vi "Shooter Simulator.vi"() -> ()   [LabVIEW 2015]
uses:
  Shooter Simulator Sensor Data.ctl
  Shooter Simulator Globals.vi
panel:
  out "R Encoder Rate":dbl
  out "L Encoder Rate":dbl
  in  "reset":bool
  out "Top Limit Switch":bool
  out "Angle Encoder Val":dbl
  out "On Fire":bool
  out "R Motor":dbl(slide) scale=-1.0..1.0
  out "L Motor":dbl(slide) scale=-1.0..1.0
  out "R RPM":dbl(knob) scale=0.0..5000.0
  out "L RPM":dbl(knob) scale=0.0..5000.0
  out "Angle Motor":dbl(slide) scale=-1.0..1.0
  out "Bottom Limit Switch":bool
  in  "Angle":dbl(slide) scale=0.0..90.0
  # "PUT ME IN PERIODIC TASKS"
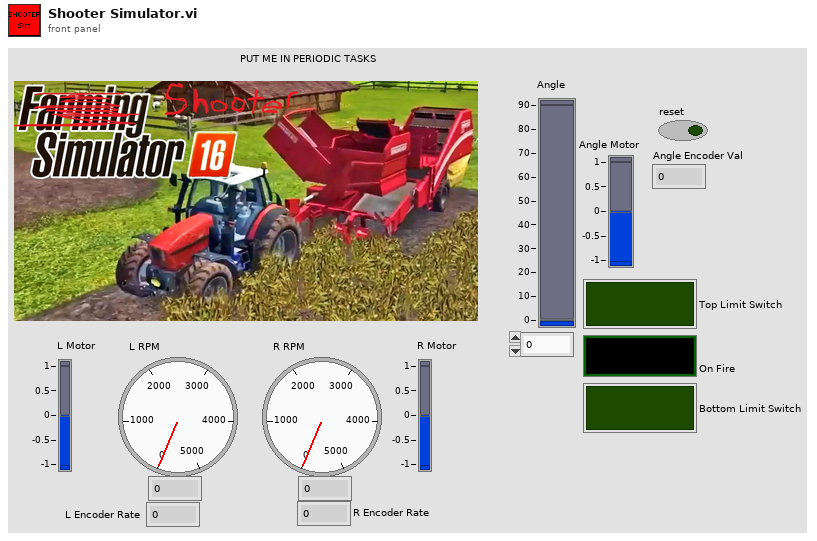
[diagram p1: front panel]
types:
  T1 = typedef "Shooter Simulator Sensor Data.ctl" = cluster{"L Enc Rate":dbl, "R Enc Rate":dbl, "Angle Encoder":dbl, "Top Limit":bool, "Bottom Limit":bool}
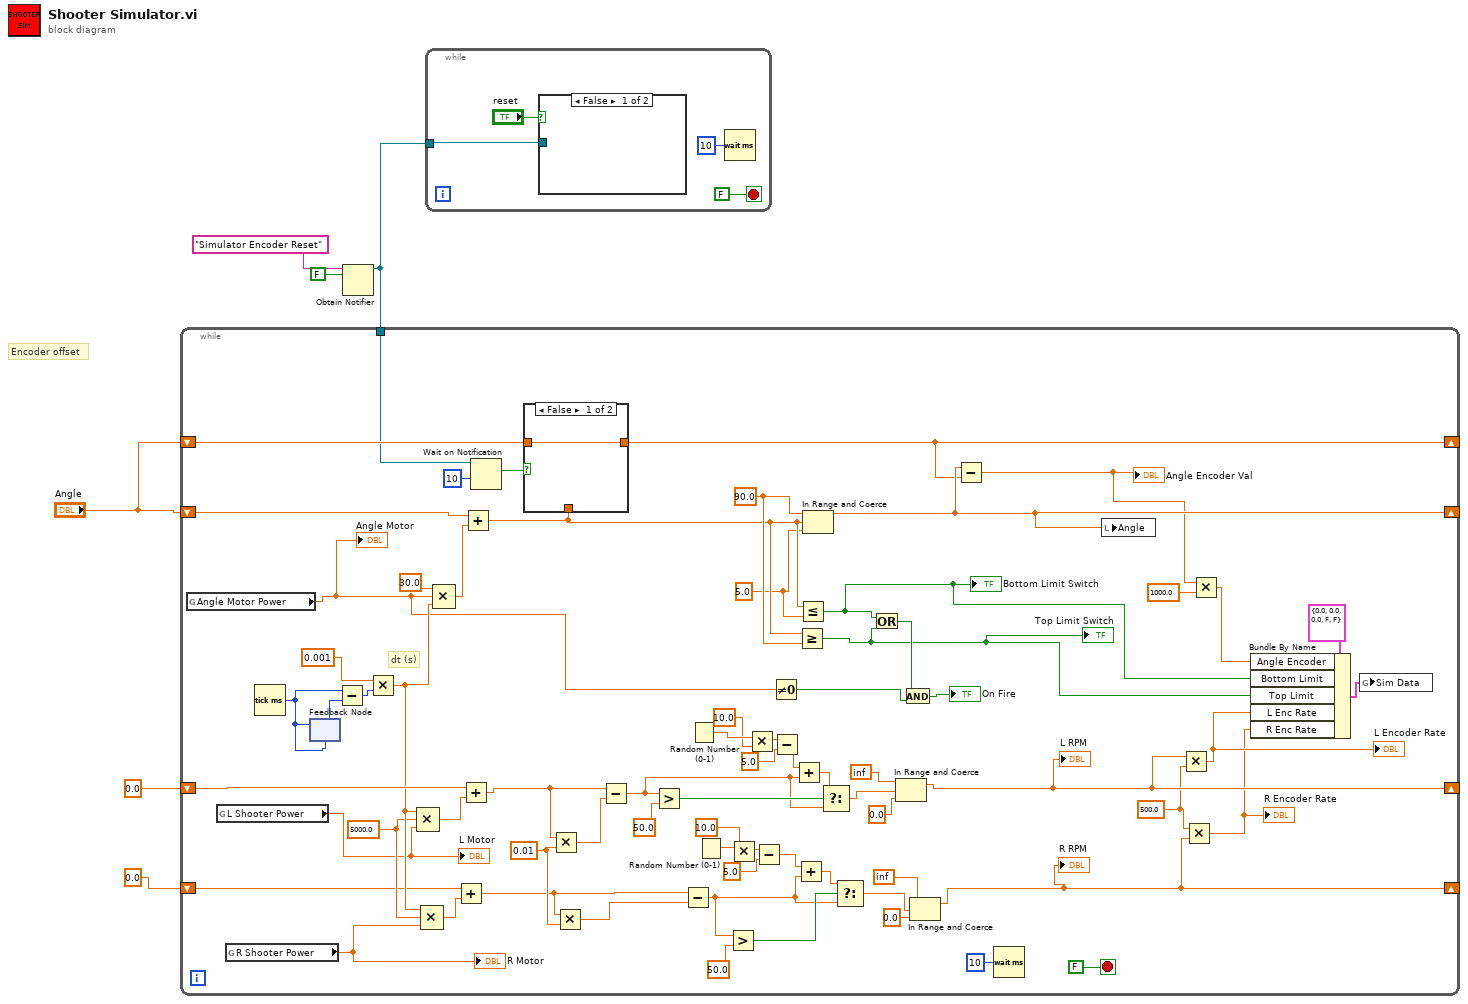
[diagram p0: block diagram]
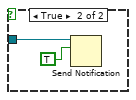
[diagram p2: hidden frame]
diagram:
  # "Encoder offset"
  n1 = Obtain Notifier(name (unnamed)="Simulator Encoder Reset", notification data type=FALSE) -> (notifier out=w2:refnum<notifier>)  [unwired: 2 in, 2 out]
  n2 = while {
    shift-right: [w63] -> _
    shift-left: "Angle" -> [w68]
    shift-right: [w64] -> _
    shift-left: "Angle" -> [w71]
    shift-right: [w18] -> _
    shift-left: 0.0 -> [w58]
    shift-right: [w19] -> _
    shift-left: 0.0 -> [w53]
    tunnel: w2 -> [w23]
    stop <- FALSE stop-if-true
    w17 = 500.0
    w51 = 0.01 ("y")
    w55 = 5000.0 ("value")
    w67 = 90.0 ("upper limit")
    w65 = 5.0 ("lower limit")
    # "dt (s)"
    n3 = global read "Shooter Simulator Globals.vi" "Angle Motor Power"() -> (w10:dbl)
    "Angle Motor" <- w10
    n4 = global read "Shooter Simulator Globals.vi" "L Shooter Power"() -> (w9:dbl)
    "L Motor" <- w9
    n5 = global read "Shooter Simulator Globals.vi" "R Shooter Power"() -> (w8:dbl)
    "R Motor" <- w8
    n6 = Tick Count (ms)() -> (millisecond timer value=w52:u32)
    n7 = feedback #1(w52) -> (w75:u32)
    n8 = feedback-in #1(w52) -> ()
    n9 = Subtract(x=w52, y=w75) -> (x-y=w74:u32)
    n10 = Multiply(x=0.001, y=w74) -> (x*y=w56:dbl)
    n11 = Compound Arithmetic op=MULTIPLY(w56, w55, w9) -> (w57:dbl)
    n12 = Compound Arithmetic op=MULTIPLY(w56, w55, w8) -> (w54:dbl)
    n13 = Compound Arithmetic op=MULTIPLY(30.0 ("value"), w10, w56) -> (w72:dbl)
    n14 = Add(x=w53, y=w54) -> (x+y=w26:dbl)
    n15 = Add(x=w58, y=w57) -> (x+y=w50:dbl)
    n16 = Add(x=w71, y=w72) -> (x+y=w66:dbl)
    n17 = Wait on Notification(notifier=w23, timeout in ms (-1)=10) -> (notification=w70:bool)  [unwired: 2 in, 3 out]
    n18 = case shown="False" w70 {
      tunnel: w68 -> [w78 _]
      tunnel: [w78 w79] -> w63
      tunnel: w66 -> [_ w79]
      frame False {
      }
      frame True {
        # "reset encoder"
      }
    }
    n19 = Multiply(x=w50, y=w51) -> (x*y=w49:dbl)
    n20 = Multiply(x=w26, y=w51) -> (x*y=w48:dbl)
    n21 = Subtract(x=w50, y=w49) -> (x-y=w30:dbl)
    n22 = Greater?(x=w30, y=50.0) -> (0:w32:bool)
    n23 = Subtract(x=w26, y=w48) -> (x-y=w7:dbl)
    n24 = Random Number (0-1)() -> (number: 0 to 1=w43:dbl)
    n25 = Random Number (0-1)() -> (number: 0 to 1=w34:dbl)
    n26 = Greater?(x=w7, y=50.0) -> (0:w24:bool)
    n27 = Multiply(x=w34, y=10.0) -> (x*y=w36:dbl)
    n28 = Multiply(x=w43, y=10.0) -> (x*y=w41:dbl)
    n29 = Subtract(x=w36, y=5.0) -> (x-y=w38:dbl)
    n30 = Not Equal To 0?(x=w10) -> (x != 0?=w62:bool)
    n31 = Subtract(x=w41, y=5.0) -> (x-y=w39:dbl)
    n32 = Add(x=w39, y=w30) -> (x+y=w31:dbl)
    n33 = Add(x=w38, y=w7) -> (x+y=w27:dbl)
    n34 = Greater Or Equal?(x=w66, y=w67) -> (x >= y?=w21:bool)
    "Top Limit Switch" <- w21
    n35 = Less Or Equal?(x=w66, y=w65) -> (x <= y?=w20:bool)
    "Bottom Limit Switch" <- w20
    n36 = In Range and Coerce(upper limit=w67, x=w66, lower limit=w65) -> (coerced(x)=w64:dbl)  [unwired: 1 out]
    n37 = Select(t=w31, s=w32, f=w30) -> (s? t:f=w29:dbl)
    n38 = Select(t=w27, s=w24, f=w7) -> (s? t:f=w28:dbl)
    n39 = Or(x=w20, y=w21) -> (x .or. y?=w61:bool)
    n40 = In Range and Coerce(upper limit=inf, x=w29, lower limit=0.0) -> (coerced(x)=w18:dbl)  [unwired: 1 out]
    "L RPM" <- w18
    n41 = And(x=w61, y=w62) -> (x .and. y?=→"On Fire":bool)
    n42 = In Range and Coerce(upper limit=inf, x=w28, lower limit=0.0) -> (coerced(x)=w19:dbl)  [unwired: 1 out]
    "R RPM" <- w19
    n43 = Subtract(x=w64, y=w63) -> (x-y=w12:dbl)
    "Angle Encoder Val" <- w12
    n44 = Wait (ms)(milliseconds to wait=u32 10) -> ()  [unwired: 1 out]
    n45 = local write "Angle"(w64) -> ()
    n46 = Multiply(x=w18, y=w17) -> (x*y=w16:dbl)
    "L Encoder Rate" <- w16
    n47 = Multiply(x=w17, y=w19) -> (x*y=w15:dbl)
    "R Encoder Rate" <- w15
    n48 = Multiply(x=w12, y=1000.0) -> (x*y=w14:dbl)
    n49 = Bundle By Name(cluster=T1 {"L Enc Rate"=0.0, "R Enc Rate"=0.0, "Angle Encoder"=0.0, "Top Limit"=FALSE, "Bottom Limit"=FALSE} ("Cluster"), "Angle Encoder"=w14, "Bottom Limit"=w20, "Top Limit"=w21, "L Enc Rate"=w16, "R Enc Rate"=w15) -> (w11:T1)
    n50 = global write "Shooter Simulator Globals.vi" "Sim Data"(w11) -> ()
  }
  n51 = while {
    tunnel: w2 -> [w82]
    stop <- FALSE stop-if-true
    n52 = case shown="False" "reset" {
      tunnel: w82 -> [_ w85]
      frame False {
      }
      frame True {
        n53 = Send Notification(notification=TRUE, notifier=w85) -> ()  [unwired: 1 in, 2 out]
      }
    }
    n54 = Wait (ms)(milliseconds to wait=u32 10) -> ()  [unwired: 1 out]
  }
